vi "SaveCSV_TXT.vi"(5 "Value":string[](array[string]), 6 "数组输入":string[](array[string]), 7 "path":path, 8 "错误输入（无错误）":errorcluster, 9 "Value 3":string[](array[string]), 10 "Value 2":i32, 11 "MulticolumnListbox输入":refnum<vi>) -> (0 "错误输出":errorcluster, 3 "MulticolumnListbox输入 2":refnum<vi>)   [LabVIEW 2018]
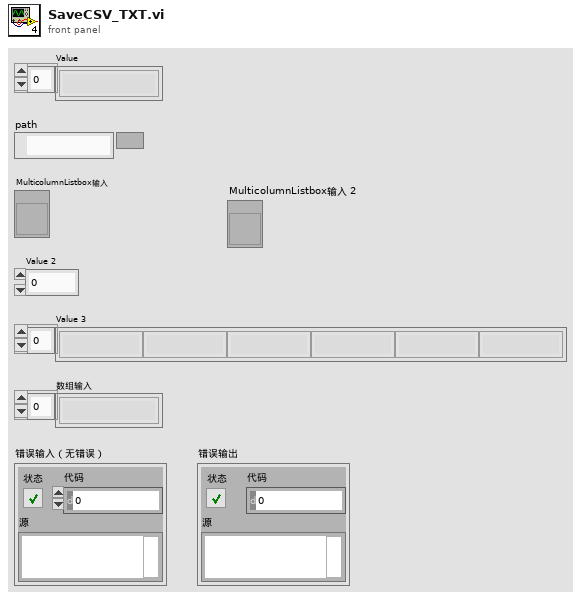
[diagram p1: front panel]
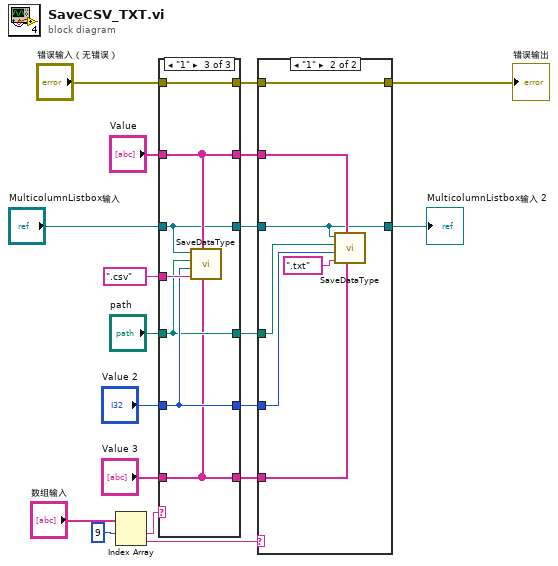
[diagram p0: block diagram]
diagram:
  n1 = Index Array(array="数组输入", index #1=9 ("索引")) -> (element #1=w10:string, element #2=w3:string)  [unwired: 1 in]
  n2 = case shown="\"1\"" w10 {
    tunnel: "Value 3" -> [w21 w27 w33]
    tunnel: "Value 2" -> [w22 w28 w36]
    tunnel: "path" -> [w23 w29 w35]
    tunnel: "MulticolumnListbox输入" -> [w24 w30 w34]
    tunnel: "Value" -> [w25 w31 w37]
    tunnel: ".csv" ("Save Type") -> [_ _ w38]
    tunnel: [w25 w31 w37] -> w11
    tunnel: [w22 w28 w36] -> w12
    tunnel: [w23 w29 w35] -> w13
    tunnel: [w24 w30 w34] -> w14
    tunnel: [w21 w27 w33] -> w15
    tunnel: [w20 w26 w32] -> w18
    tunnel: "错误输入（无错误）" -> [w20 w26 w32]
    frame "假", Default {
    }
    frame "0" {
    }
    frame "1" {
      n3 = call "SaveDataType.vi"("Value 3"=w33, "Value 2"=w37, "Save Type"=w38, "Value"=w36, "path"=w35, "MulticolumnListbox输入"=w34) -> ()  [unwired: 5 in, 1 out]
    }
  }
  n4 = case shown="\"1\"" w3 {
    tunnel: w15 -> [_ w46]
    tunnel: w12 -> [_ w45]
    tunnel: w13 -> [_ w44]
    tunnel: w14 -> [w39 w41]
    tunnel: w11 -> [_ w43]
    tunnel: [w40 w42] -> w17
    tunnel: w18 -> [w40 w42]
    tunnel: [w39 w41] -> w1
    frame "假", Default {
    }
    frame "1" {
      n5 = call "SaveDataType.vi"("Value 3"=w46, "Value 2"=w43, "Save Type"=".txt", "Value"=w45, "path"=w44, "MulticolumnListbox输入"=w41) -> ()  [unwired: 5 in, 1 out]
    }
  }
  "错误输出" <- w17
  "MulticolumnListbox输入 2" <- w1
